vi "Data_Display_global.vi"() -> ()   [LabVIEW 2016]
uses:
  Monitors/Utility/Monitor Communication/Gustav/20TVTI_Cluster.ctl
  Monitors/Utility/Monitor Communication/Gustav/20T_Cluster.ctl
  Monitors/Utility/Monitor Communication/JT/JT-Status-DD.ctl
  Monitors/Equipment/LS370_Status.ctl
  Monitors/Utility/Monitor Communication/S16/VTI-cluster.ctl
  Monitors/Utility/Monitor Communication/LS350/LS350-cluster.ctl
  Monitors/Utility/Monitor Communication/S16/16T-Cluster.ctl
  Monitors/Utility/Monitor Communication/SR830/SR830-Cluster.ctl
  Monitors/Utility/Monitor Communication/S16/ILM-Cluster.ctl
  Monitors/Utility/Monitor Communication/Gustav/20T_Dewar_Cluster.ctl
panel:
  in  "20T-Dewar-Cluster":T1={"Dewar Heater (%)"=0.0, "D-Heater (%) Display"=3.4572, "D-Heater SP"=0.0, "Set D-Heater SP"=FALSE, "Change D-Heater Status"=FALSE, "Dewar Pressure"=0.0, "Dewar heater manual"=FALSE} {"Dewar Pressure" format="%4_5f"; "D-Heater (%) Display" format="%4_5f"; "Dewar Heater (%)" scale=0.0..100.0}
  out "ILM":T2 {"Nitrogen" format="%#4_5f"}
  out "SR830-1":T3={"Lockin 1"=[], "X1"=0.0, "Y1"=0.0, "X1 Percent"=0.0, "X1 Overload"=FALSE, "Y1 Overload"=FALSE, "Unit X1"="nV", "Unit X2"="nV", "Unit X2a"="nV", "Unit X1a"="nV", "Sensitivity Setpoint"=26, "X1 Percent 2"=0.0} {"X1 Percent 2" scale=0.0..1.0; "Sensitivity Setpoint" items=["2 nV", "5 nV", "10 nV", "20 nV", "50 nV", "100 nV", "200 nV", "500 nV", "1 µV", "2 µV", "5 µV", "10 µV", "20 µV", "50 µV", "100 µV", "200 µV", "500 µV", "1 mV", "2 mV", "5 mV", "10 mV", "20 mV", "50 mV", "100 mV", "200 mV", "500 mV", "1 V", ""]; "X1 Percent" scale=0.0..1.0; "X1" format="%#4_5f"}
  out "SR830-2":T3={"Lockin 1"=[], "X1"=0.0, "Y1"=0.0, "X1 Percent"=0.0, "X1 Overload"=FALSE, "Y1 Overload"=FALSE, "Unit X1"="nV", "Unit X2"="nV", "Unit X2a"="nV", "Unit X1a"="nV", "Sensitivity Setpoint"=26, "X1 Percent 2"=0.0} {"X1 Percent 2" scale=0.0..1.0; "Sensitivity Setpoint" items=["2 nV", "5 nV", "10 nV", "20 nV", "50 nV", "100 nV", "200 nV", "500 nV", "1 µV", "2 µV", "5 µV", "10 µV", "20 µV", "50 µV", "100 µV", "200 µV", "500 µV", "1 mV", "2 mV", "5 mV", "10 mV", "20 mV", "50 mV", "100 mV", "200 mV", "500 mV", "1 V", ""]; "X1 Percent" scale=0.0..1.0; "X1" format="%#4_5f"}
  in  "16 T Cluster":T4={"Clamp"=FALSE, "Switch Heater"=FALSE, "Go to Zero"=FALSE, "Go to set"=FALSE, "Go to Hold"=FALSE, "Clamped"=FALSE, "Quenched"=FALSE, "Rate limit"=FALSE, "Persistent"=FALSE, "Hold"=FALSE, "Set"=FALSE, "Zero"=FALSE, "Magnet (T)"=0.0, "Leads (T)"=0.0, "Magnet T (K)"=3.4572, "Switch"=FALSE, "Setpoint (T)"=3.4572, "Rate (T/min)"=0.0, "Select"=FALSE, "Sweeping"=FALSE} caption="16 T Magnet control" {"Rate (T/min)" format="%6_5f"; "Setpoint (T)" format="%6_5f"; "Magnet T (K)" format="%#4_5f"; "Leads (T)" format="%6_5f"}
  in  "Lakeshore 350":T5 {"Setpoint control" format="%6_5f"}
  out "VTI Sweep Running":bool
  out "Current VTI Setpoint":dbl
  in  "VTI":T6={"Temperatur (K)"=0.0, "Setpoint (K)"=0.0, "Rate (K/min)"=3.4572, "Heater (%)"=0.0, "NV (%)"=0.0, "Heater Manual"=FALSE, "NV Manual"=FALSE, "Go to Set"=FALSE, "Pressure"=0.0, "Heater SP"=0.0, "Valid?"=FALSE, "Set Heater SP"=FALSE, "Set NV SP"=FALSE, "Heater (%) Display"=3.4572, "NV (%) Display"=3.4572, "NV Setpoint"=0.0, "Change Heater Status"=FALSE, "Change NV Status"=FALSE, "Sample 3"=0.0, "Sample 2"=0.0, "Sweep-State"=FALSE, "Set Auto PID"=FALSE, "Auto PID"=FALSE, "Stopp"=FALSE, "Setpoint-Sweep"=0.0} {"NV (%) Display" format="%4_5f"; "Heater (%) Display" format="%4_5f"; "Pressure" format="%#4_5f"; "NV (%)" scale=0.0..100.0; "Heater (%)" scale=0.0..100.0; "Rate (K/min)" format="%#4_5f"; "Setpoint (K)" format="%6_5f"}
  out "Critical Error":bool
  out "Lakeshore 370":T7
  in  "JT-Cluster":T8 {"Dump" scale=0.0..100.0}
  out "20 T Magnet control":T9={"Clamp"=FALSE, "Switch Heater"=FALSE, "Go to Zero"=FALSE, "Go to set"=FALSE, "Go to Hold"=FALSE, "Clamped"=FALSE, "Quenched"=FALSE, "Rate limit"=FALSE, "Persistent"=FALSE, "Hold"=FALSE, "Set"=FALSE, "Zero"=FALSE, "Magnet (T)"=0.0, "Leads (T)"=0.0, "Magnet T (K)"=3.4572, "Switch"=FALSE, "Target (T)"=3.4572, "Setpoint (T)"=3.4572, "Rate (T/min)"=0.0, "Switch Heater 2"=FALSE, "Set Rate"=FALSE} {"Rate (T/min)" format="%6_5f"; "Setpoint (T)" format="%6_5f"; "Target (T)" format="%#4_5f"; "Magnet T (K)" format="%#4_5f"; "Leads (T)" format="%6_5f"}
  out "Monitor Start":timestamp
  in  "20TVTI":T10={"Temperatur (K)"=0.0, "Setpoint (K)"=0.0, "Rate (K/min)"=3.4572, "Heater (%)"=0.0, "NV (%)"=0.0, "Heater Manual"=FALSE, "NV Manual"=FALSE, "Go to Set"=FALSE, "Pressure"=0.0, "Heater SP"=0.0, "Valid?"=FALSE, "Set Heater SP"=FALSE, "Set NV SP"=FALSE, "Heater (%) Display"=3.4572, "NV (%) Display"=3.4572, "NV Setpoint"=0.0, "Change Heater Status"=FALSE, "Change NV Status"=FALSE, "Change Sweep Type"=FALSE} {"NV (%) Display" format="%4_5f"; "Heater (%) Display" format="%4_5f"; "Heater SP" format="%4_5f"; "Pressure" format="%#4_5f"; "NV (%)" scale=0.0..100.0; "Heater (%)" scale=0.0..100.0; "Rate (K/min)" format="%#4_5f"; "Setpoint (K)" format="%6_5f"}
  in  "Switch Button Text":string
  out "Error":bool
  in  "Error String":string
  out "Dewar Pressure (mbar)":dbl
  out "recondense - heat (%)":dbl
  out "Z Axis Status":T11(ring)=enum."RAMPING"
  out "Y Axis Status":T11(ring)=enum."RAMPING"
  out "AMI Set field":bool
  out "AMI Set field rates":bool
  out "Switch Heater On":bool
  out "Switch Heater Z":bool
  out "B AMI rate (T)":dbl
  out "Phi AMI Setpoint (Deg)":dbl
  out "B AMI Setpoint (T)":dbl
  out "Phi AMI (Deg)":dbl
  out "B AMI (T)":dbl
  out "AMI Monitor":bool
  out "Z-Axis Rate (T/min)":dbl
  out "Y-Axis Rate (T/min)":dbl
  out "Z-Axis Setpoint (T)":dbl
  out "Y-Axis Setpoint (T)":dbl
  out "Switch Heater Y":bool
  out "Z-Axis (T)":dbl
  out "Y-Axis (T)":dbl
  out "Offset 6221":dbl
  out "Offset Setp 6221":dbl
  out "End of measurement":timestamp
  out "Keithley 6221 Compl":bool
  out "Frequency Setp 6221":dbl=1000.0
  out "Keithley 6221\nOutput ON/OFF":bool
  out "Keithley 6221 Output Status":bool
  out "Set Keithley 6221":bool
  out "LS340 Heater ON/OFF":bool
  in  "LS340 Heater":dbl
  out "Set Keithley Output":bool
  out "Keithley Output Status":bool
  out "Keithley Current Setpoint":dbl
  out "Set Current":bool
  out "Frequency 6221":dbl
  out "Amplitude Setp 6221":dbl
  out "Amplitude 6221":dbl
  out "Rate":bool
  out "Slow":bool
  out "Fast":bool
  out "Set LNV - Bool":bool
  in  "Set LNV":dbl
  out "Lambda Pressure":dbl
  out "Lambda NV":dbl
  in  "Last reading":dbl
  out "Update AH":bool
  in  "End of row":string
  in  "Remaining Duration of rows":string
  in  "Remaining Duration":string
  out "Sensitivity Setpoint 3":i32
  out "Sensitivity Setpoint 2":i32
  out "Sensitivity Setpoint 1":i32
  out "Datafile-Counter":dbl=10000.0
  out "Select":bool
  out "Confirm":bool
  out "Zero":bool
  out "Set":bool
  out "Persistent":bool
  out "Rate limit":bool
  out "Quenched":bool
  out "Clamped":bool
  out "Hold":bool
  out "Magnet T (K)":dbl
  out "Nitrogen(%)":dbl=99.4
  out "Helium (%)":dbl=63.1
  out "Switch heater waiting":bool
  out "Sens Ovl 3":bool
  out "Sens Ovl 2":bool
  out "Sens Ovl 1":bool
  out "Switch Heater waiting time":dbl
  out "Res Keithley 4R":dbl
  in  "Stop Monitors":bool
  out "Sensitivity 3":i32
  out "Y3":dbl
  out "X3":dbl
  out "Sensitivity 2":i32
  out "Sensitivity 1":i32
  out "Y2":dbl
  out "X2":dbl
  out "Y1":dbl
  out "X1":dbl
  out "Loss":dbl
  out "Capacity":dbl
  out "LS372-R6":dbl
  out "LS372-R5":dbl
  out "LS372-T6":dbl
  out "LS372-T5":dbl
  out "Control Temperature Resistance":dbl
  out "LS372-R4":dbl
  out "LS372-R3":dbl
  out "LS372-T4":dbl
  out "LS372-T3":dbl
  out "LS372-R2":dbl
  out "LS372-R1":dbl
  out "LS372 -T2":dbl
  out "LS372-T1":dbl
  out "Sorb Temperature":dbl
  out "Still Res":dbl
  out "Still Temp":dbl
  out "Angle Step Sweep":bool
  out "Lock In 3 Channel 2":dbl
  out "Lock In 3 Channel 1":dbl
  out "Angle":dbl
  out "current angle setpoint":dbl
  out "current temperature setpoint":dbl
  out "Sample Temperature Lakeshore 340":dbl
  out "current I setpoint":dbl
  out "Voltage":dbl
  out "Resistance":dbl
  out "Current":dbl
  out "CC running time":dbl
  out "waiting time":dbl
  out "current number of steps":i32
  out "current field setpoint":dbl
  out "B_final reached":bool
  out "B_init reached":bool
  out "T_final reached":bool
  out "T_init reached":bool
  out "Lock In 2 Channel 2":dbl
  out "Lock In 2 Channel 1":dbl
  out "Lock In 1 Channel 2":dbl
  out "Lock In 1 Channel 1":dbl
  out "Magnetic Field SC":dbl
  out "Magnetic Field Init":dbl
  out "Sample Temperature 2 SC":dbl
  out "Sample Temperature 1 SC":dbl
  out "Control Temperature SC":dbl
  out "Control Temperature Init":dbl
  out "Init/SC Selector":bool
  # "ILM & Lambda Stage"
  # "Timing"
  # "IPS"
  # "Lakeshore 370"
  # "AH 2700A"
  # "Keithely 4R"
  # "Temperature"
  # "Resistance"
  # "SR 830"
  # "Time Data Write"
  # "Lockin 1"
  # "Lakeshore 372"
  # "Temperature"
  # "Resistance"
  # "Keithely"
  # "Keithely 6221"
  # "LS340 Control"
  # "Lockin 2"
  # "Lockin 3"
  # "AMI Control YZ Axis Magnet"
  # "Dewar Heater (%)"
  # "Dewar Pressure"
  # "Setpoint"
  # "20T Dewar"
  # "N (%)"
  # "He (%)"
  # "Levelmeter"
  # "SR830-1"
  # "SR830-2"
  # "Dill. unit"
  # "LN2\nTrap"
  # "12"
  # "15"
  # "20 T"
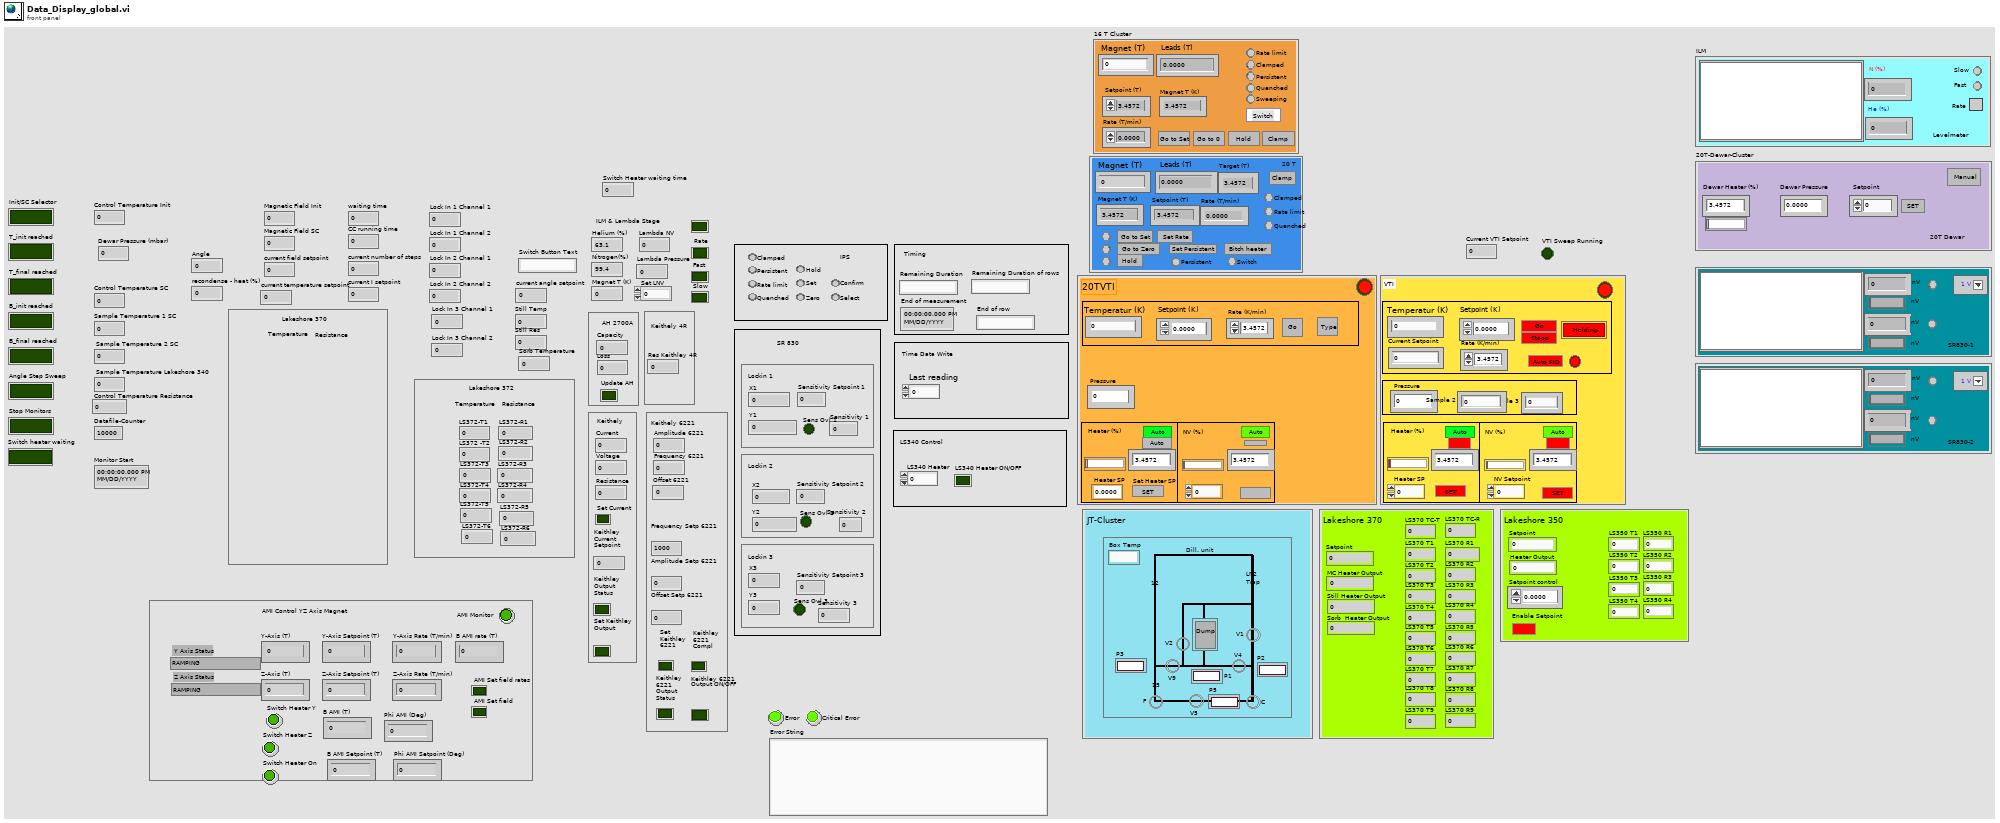
[diagram p1: front panel]
types:
  T1 = typedef "20T_Dewar_Cluster.ctl" = cluster{"Dewar Heater (%)":dbl, "D-Heater (%) Display":dbl, "D-Heater SP":dbl, "Set D-Heater SP":bool, "Change D-Heater Status":bool, "Dewar Pressure":dbl, "Dewar heater manual":bool}
  T2 = typedef "ILM-Cluster.ctl" = cluster{"Plot":dbl[][], "Nitrogen":dbl, "Helium":dbl, "Fast":bool, "Slow":bool, "Rate":bool}
  T3 = typedef "SR830-Cluster.ctl" = cluster{"Lockin 1":dbl[][], "X1":dbl, "Y1":dbl, "X1 Percent":dbl, "X1 Overload":bool, "Y1 Overload":bool, "Unit X1":string, "Unit X2":string, "Unit X2a":string, "Unit X1a":string, "Sensitivity Setpoint":i16, "X1 Percent 2":dbl}
  T4 = typedef "16T-Cluster.ctl" = cluster{"Clamp":bool, "Switch Heater":bool, "Go to Zero":bool, "Go to set":bool, "Go to Hold":bool, "Clamped":bool, "Quenched":bool, "Rate limit":bool, "Persistent":bool, "Hold":bool, "Set":bool, "Zero":bool, "Magnet (T)":dbl, "Leads (T)":dbl, "Magnet T (K)":dbl, "Switch":bool, "Setpoint (T)":dbl, "Rate (T/min)":dbl, "Select":bool, "Sweeping":bool}
  T5 = typedef "LS350-cluster.ctl" = cluster{"Setpoint":dbl, "Heater Output":dbl, "Setpoint control":dbl, "Enable Setpoint":bool, "LS350 T1":dbl, "LS350 T2":dbl, "LS350 T3":dbl, "LS350 T4":dbl, "LS350 R1":dbl, "LS350 R2":dbl, "LS350 R3":dbl, "LS350 R4":dbl}
  T6 = typedef "VTI-cluster.ctl" = cluster{"Temperatur (K)":dbl, "Setpoint (K)":dbl, "Rate (K/min)":dbl, "Heater (%)":dbl, "NV (%)":dbl, "Heater Manual":bool, "NV Manual":bool, "Go to Set":bool, "Pressure":dbl, "Heater SP":dbl, "Valid?":bool, "Set Heater SP":bool, "Set NV SP":bool, "Heater (%) Display":dbl, "NV (%) Display":dbl, "NV Setpoint":dbl, "Change Heater Status":bool, "Change NV Status":bool, "Sample 3":dbl, "Sample 2":dbl, "Sweep-State":bool, "Set Auto PID":bool, "Auto PID":bool, "Stopp":bool, "Setpoint-Sweep":dbl}
  T7 = typedef "LS370_Status.ctl" = cluster{"Setpoint":dbl, "MC Heater Output":dbl, "Still Heater Output":dbl, "Sorb  Heater Output":dbl, "LS370 T1":dbl, "LS370 T2":dbl, "LS370 T3":dbl, "LS370 T4":dbl, "LS370 T5":dbl, "LS370 R1":dbl, "LS370 R2":dbl, "LS370 R3":dbl, "LS370 R4":dbl, "LS370 R5":dbl, "LS370 T6":dbl, "LS370 T7":dbl, "LS370 T8":dbl, "LS370 T9":dbl, "LS370 R6":dbl, "LS370 R7":dbl, "LS370 R8":dbl, "LS370 R9":dbl, "LS370 TC-T":dbl, "LS370 TC-R":dbl}
  T8 = typedef "JT-Status-DD.ctl" = cluster{"V2":bool, "V5":bool, "V1":bool, "V9":bool, "F":bool, "C":bool, "V4":bool, "Dump":u8, "P3":dbl, "P1":dbl, "P2":dbl, "P5":dbl, "Box Temp":dbl}
  T9 = typedef "20T_Cluster.ctl" = cluster{"Clamp":bool, "Switch Heater":bool, "Go to Zero":bool, "Go to set":bool, "Go to Hold":bool, "Clamped":bool, "Quenched":bool, "Rate limit":bool, "Persistent":bool, "Hold":bool, "Set":bool, "Zero":bool, "Magnet (T)":dbl, "Leads (T)":dbl, "Magnet T (K)":dbl, "Switch":bool, "Target (T)":dbl, "Setpoint (T)":dbl, "Rate (T/min)":dbl, "Switch Heater 2":bool, "Set Rate":bool}
  T10 = typedef "20TVTI_Cluster.ctl" = cluster{"Temperatur (K)":dbl, "Setpoint (K)":dbl, "Rate (K/min)":dbl, "Heater (%)":dbl, "NV (%)":dbl, "Heater Manual":bool, "NV Manual":bool, "Go to Set":bool, "Pressure":dbl, "Heater SP":dbl, "Valid?":bool, "Set Heater SP":bool, "Set NV SP":bool, "Heater (%) Display":dbl, "NV (%) Display":dbl, "NV Setpoint":dbl, "Change Heater Status":bool, "Change NV Status":bool, "Change Sweep Type":bool}
  T11 = enum16{"", "RAMPING", "HOLDING", "PAUSED", "MANUAL UP", "MANUAL DOWN", "ZEROING CURRENT", "QUENCH DETECTED", "HEATING SWITCH", "AT ZER0", "COOLING SWITCH"}
diagram:
